vi "Actor Core.vi"(8 "error in":errorcluster, 11 "NI in":refnum<class "NI.lvclass">) -> (0 "error out":errorcluster, 3 "Actor out":refnum<class "Actor.lvclass">)   [LabVIEW 2021, in "NI.lvlib" / "NI.lvclass"]
doc: "(<B>Filename</B>: Actor Framework.lvlib:Actor.lvclass:Actor Core.vi)\n\nReceives messages to the actor, reacts to them, and initiates any error handling that may shut the actor down.\n\nDescendant classes may override this VI to append parallel tasks for the actor to complete while it handles messages. Overrides use the Call Parent Method node."
uses:
  NI.lvclass
  C:/Program Files (x86)/National Instruments/LabVIEW 2021/vi.lib/ActorFramework/Actor/Actor.lvclass
  <vilib>/ActorFramework/Actor/Actor.lvclass
  NI.lvclass/NI.ctl
  <vilib>/ActorFramework/Actor/Actor.lvclass/Actor.ctl
  <vilib>/ActorFramework/Message Enqueuer/Message Enqueuer.lvclass/Message Enqueuer.ctl
  <vilib>/ActorFramework/Message Enqueuer/Message Priority.ctl
  NI Messages/NI change z offset Msg/NI change z offset Msg.lvclass/NI change z offset Msg.ctl
  <vilib>/ActorFramework/Message Enqueuer/Init from Existing Queue.vi
  <vilib>/ActorFramework/Message Enqueuer/Enqueue.vi
  NI Messages/NI update wav display Msg/NI update wav display Msg.lvclass
  C:/Program Files (x86)/National Instruments/LabVIEW 2021/vi.lib/ActorFramework/Message/Message.lvclass
  NI Messages/NI change inner param Msg/NI change inner param Msg.lvclass
  NI Messages/NI change z offset Msg/NI change z offset Msg.lvclass
  <vilib>/ActorFramework/Message Priority Queue/Priority Enqueue.vi
  <vilib>/ActorFramework/Message Enqueuer/Message Enqueuer.lvclass
panel:
  in  "Offset":dbl(slide)=5.0 min=-5.0 max=5.0 step=0.0066 scale=-1.0..1.0
  in  "Open Connection":bool
  in  "Auto update?":bool
  out "Waveform Graph":dbl[](graph)
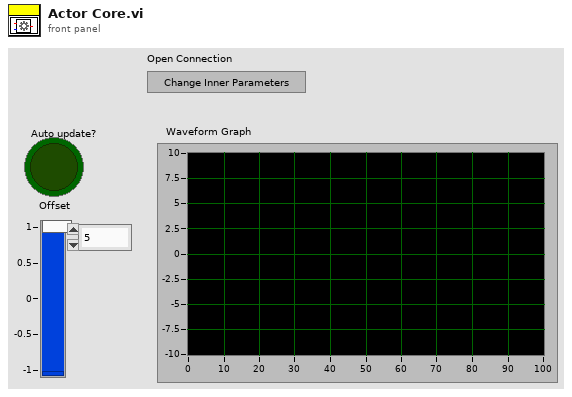
[diagram p1: front panel]
types:
  T1 = typedef "Actor Framework.lvlib/Message Enqueuer.lvclass/Message Priority.ctl" = enum16{"Low", "Normal", "High"}
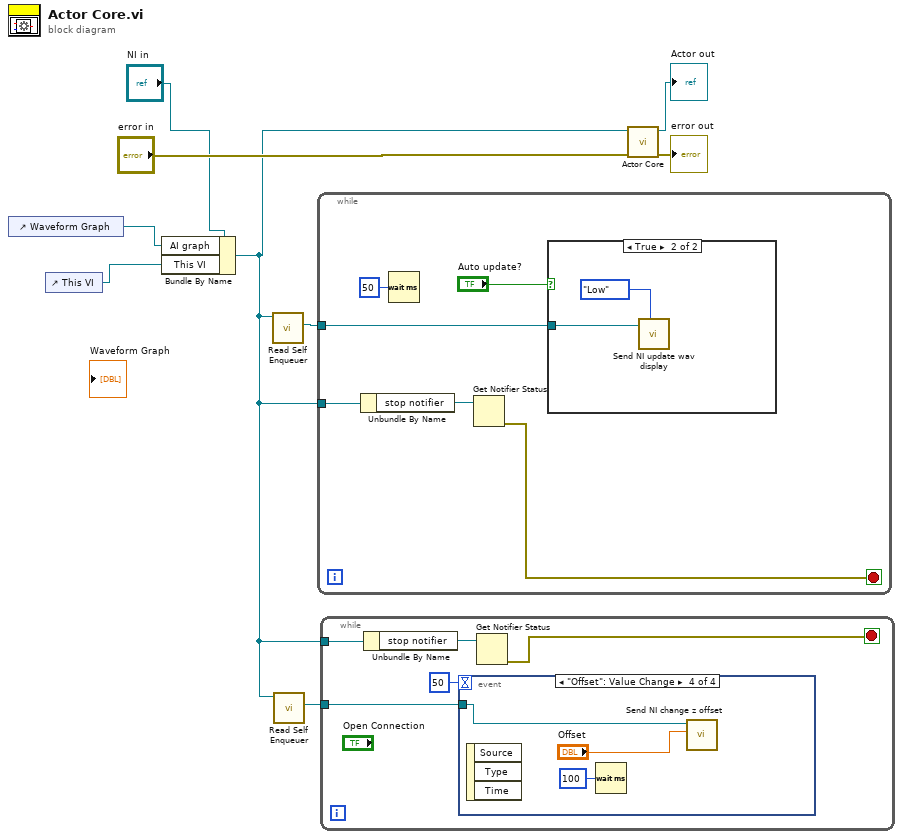
[diagram p0: block diagram]
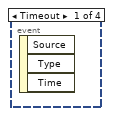
[diagram p2: hidden frame]
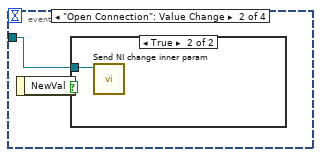
[diagram p3: hidden frame]
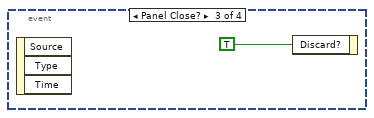
[diagram p5: hidden frame]
diagram:
  n1 = control-ref of="Waveform Graph"() -> (w5:refnum<vi>)
  n2 = control-ref of="This VI"() -> (w4:refnum<vi>)
  n3 = Bundle By Name(cluster="NI in", "AI graph"=w5, "This VI"=w4) -> (w2:refnum<class "NI.lvclass">)
  n4 = call <vilib>:"Read Self Enqueuer.vi"("Actor"=w2) -> ("Self Enqueuer"=w3:refnum<class "Message Enqueuer.lvclass">)  [unwired: 10 in]
  n5 = call <vilib>:"Read Self Enqueuer.vi"("Actor"=w2) -> ("Self Enqueuer"=w1:refnum<class "Message Enqueuer.lvclass">)  [unwired: 10 in]
  n6 = while {
    tunnel: w2 -> [w14]
    tunnel: w3 -> [w11]
    stop <- w12 stop-if-true
    n7 = Unbundle By Name(w14) -> ("stop notifier"=w13:refnum<notifier>)
    n8 = Wait (ms)(milliseconds to wait=u32 50) -> ()  [unwired: 1 out]
    n9 = Get Notifier Status(notifier=w13) -> (error out=w12:errorcluster)  [unwired: 1 in, 4 out]
    n10 = case shown="True" "Auto update?" {
      tunnel: w11 -> [_ w16]
      frame False {
      }
      frame True {
        n11 = call "Send NI update wav display.vi"("Message Priority (Normal)"=Message_Priority."Low", "Message Enqueuer"=w16) -> ()  [unwired: 8 in, 2 out]
      }
    }
  }
  n12 = while {
    tunnel: w2 -> [w22]
    tunnel: w1 -> [w19]
    stop <- w20 stop-if-true
    n13 = Unbundle By Name(w22) -> ("stop notifier"=w21:refnum<notifier>)
    n14 = event shown="[3] \"Offset\": Value Change" {
      selector: _ -> [_ _ _ _]
      dyn-events: _ -> [_ _ _ _]
      timeout: 50 -> [_ _ _ _]
      tunnel: w19 -> [_ w24 _ w28]
      event Timeout {
        n15 = event-data() -> ()  [unwired: 1 in, 3 out]
      }
      event "Open Connection": Value Change {
        n16 = event-data() -> ("NewVal"=w23:bool)  [unwired: 1 in]
        n17 = case shown="True" w23 {
          tunnel: w24 -> [_ w25]
          frame False {
          }
          frame True {
            n18 = call "Send NI change inner param.vi"("Message Enqueuer"=w25) -> ()  [unwired: 9 in, 2 out]
          }
        }
      }
      event Panel Close? {
        n19 = event-data() -> ()  [unwired: 1 in, 3 out]
        n20 = event-data("Discard?"=TRUE) -> ()  [unwired: 1 in, 1 out]
      }
      event "Offset": Value Change {
        n21 = event-data() -> ()  [unwired: 1 in, 3 out]
        n22 = Wait (ms)(milliseconds to wait=u32 100) -> ()  [unwired: 1 out]
        n23 = call "Send NI change z offset.vi"("offset"="Offset", "Message Enqueuer"=w28) -> ()  [unwired: 8 in, 2 out]
      }
    }
    n24 = Get Notifier Status(notifier=w21) -> (error out=w20:errorcluster)  [unwired: 1 in, 4 out]
  }
  n25 = call-parent "Actor Core.vi"("error in"="error in", "Actor in"=w2) -> ("error out"=→"error out":errorcluster, "Actor out"=→"Actor out":refnum<class "Actor.lvclass">)  [unwired: 8 in]
